vi "Modbus Visa for Solder.vi"(1 "VISA resource name":refnum<visa-resource-name>, 2 "Cmd":string, 3 "TimeOut":bool=TRUE, 4 "Time(0.1)":u32=10, 5 "error in (no error)":errorcluster, 8 "VisaAction":T1(ring)) -> (16 "read string":string, 19 "error out":errorcluster)   [LabVIEW 2019]
uses:
  <vilib>/Instr/_visa.llb/VISA Configure Serial Port (Instr).vi
panel:
  in  "TimeOut 2":bool=TRUE
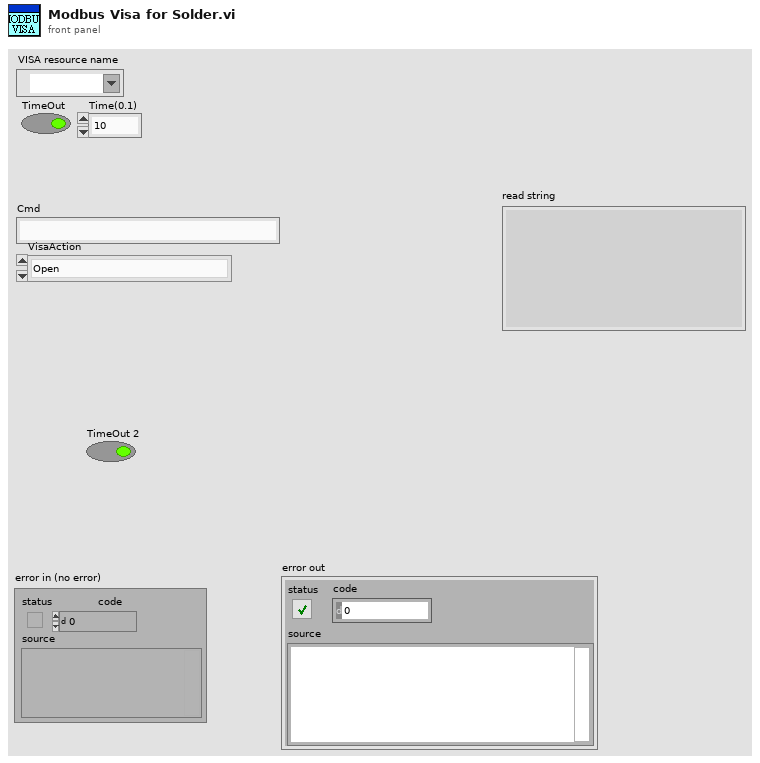
[diagram p1: front panel]
types:
  T1 = enum16{"Open", "Send", "Recieve", "Recieve cmd", "Close"}
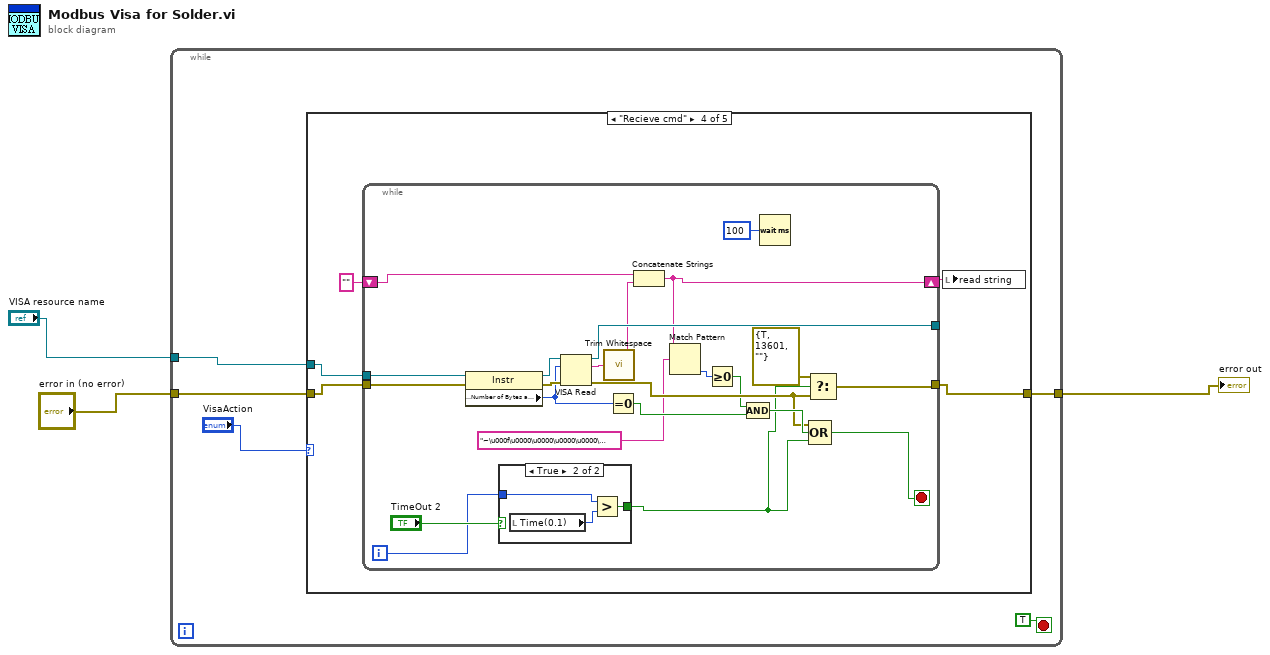
[diagram p0: block diagram]
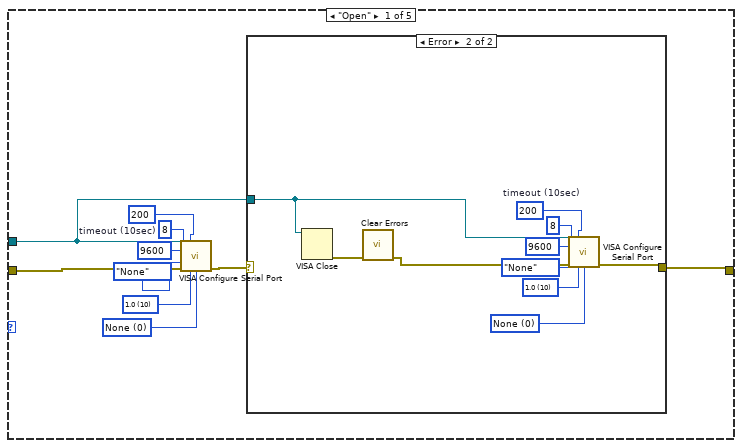
[diagram p2: hidden frame]
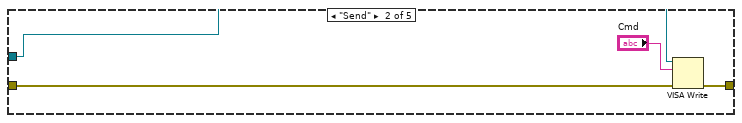
[diagram p4: hidden frame]
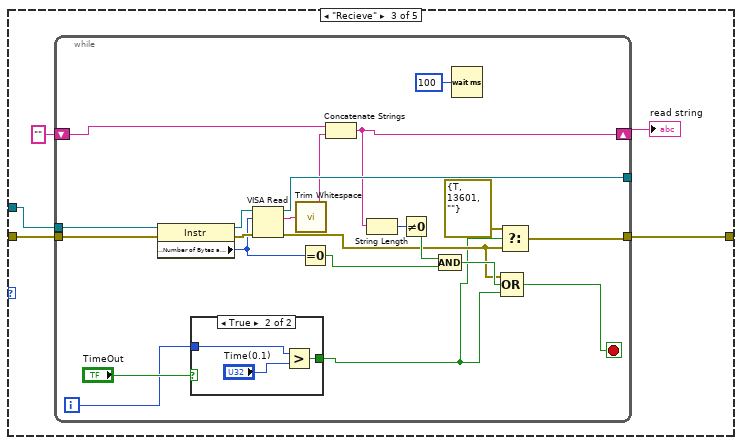
[diagram p5: hidden frame]
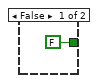
[diagram p6: hidden frame]
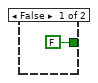
[diagram p7: hidden frame]
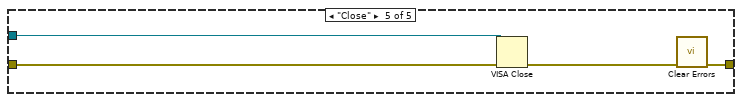
[diagram p8: hidden frame]
diagram:
  n1 = while {
    tunnel: "error in (no error)" -> [w7]
    tunnel: [w8] -> w3
    tunnel: "VISA resource name" -> [w5]
    stop <- TRUE stop-if-true
    n2 = case shown="\"Recieve cmd\"" "VisaAction" {
      tunnel: [w10 w33 w37 w67 w98] -> w8
      tunnel: w7 -> [w18 w32 w38 w65 w99]
      tunnel: w5 -> [w9 w31 w34 w66 w97]
      frame "Open" {
        w13 = u16 0 items=["None", "XON/XOFF", "RTS/CTS", "XON/XOFF & RTS/CTS", "DTR/DSR", "XON/XOFF & DTR/DSR"] ("flow control (0:none)")
        w14 = u16 10 items=["1.0"=10, "1.5"=15, "2.0"=20] ("stop bits (10: 1 bit)")
        w17 = u32 200  # timeout (10sec)
        n3 = call-poly "VISA Configure Serial Port"("VISA resource name"=w9, "timeout (10sec)"=w17, "baud rate (9600)"=u32 9600, "data bits (8)"=u16 8, "parity (0:none)"=enum16{"None", "Odd", "Even", "Mark", "Space"}."None", "error in (no error)"=w18, "stop bits (10: 1 bit)"=w14, "flow control (0:none)"=w13) -> ("error out"=w11:errorcluster)  [unwired: 1 in, 6 out]
        n4 = case shown="Error" w11 {
          selector: w11 -> [w19 _]
          tunnel: [w19 w20] -> w10
          tunnel: w9 -> [_ w21]
          frame No Error {
          }
          frame Error {
            w28 = u16 0 items=["None", "XON/XOFF", "RTS/CTS", "XON/XOFF & RTS/CTS", "DTR/DSR", "XON/XOFF & DTR/DSR"] ("flow control (0:none)")
            w27 = u16 10 items=["1.0"=10, "1.5"=15, "2.0"=20] ("stop bits (10: 1 bit)")
            w24 = u32 200  # timeout (10sec)
            n5 = VISA Close(VISA resource name=w21) -> (error out=w23:errorcluster)  [unwired: 1 in]
            n6 = call <vilib>:"Clear Errors.vi"("error in (no error)"=w23) -> ("error out"=w22:errorcluster)  [unwired: 5 in, 1 out]
            n7 = call-poly "VISA Configure Serial Port"("VISA resource name"=w21, "timeout (10sec)"=w24, "baud rate (9600)"=u32 9600, "data bits (8)"=u16 8, "parity (0:none)"=enum16{"None", "Odd", "Even", "Mark", "Space"}."None", "error in (no error)"=w22, "stop bits (10: 1 bit)"=w27, "flow control (0:none)"=w28) -> ("error out"=w20:errorcluster)  [unwired: 1 in, 6 out]
          }
        }
      }
      frame "Send" {
        n8 = VISA Write(VISA resource name=w31, write buffer="Cmd", error in (no error)=w32) -> (error out=w33:errorcluster)  [unwired: 2 out]
      }
      frame "Recieve" {
        n9 = while {
          tunnel: w38 -> [w58]
          tunnel: [w57] -> _
          tunnel: [w52] -> w37
          shift-right: [w49] -> w36
          shift-left: "" ("trimmed string") -> [w55]
          tunnel: w34 -> [w39]
          i -> [w41]
          stop <- w53 stop-if-true
          n10 = property class="Instr"(reference=w39, error in=w58) -> (reference out=w59:refnum<visa-resource-name>, error out=w60:errorcluster, "Serial Settings:Number of Bytes at Serial Port"=w42:u32)
          n11 = case shown="True" "TimeOut" {
            tunnel: w41 -> [_ w64]
            tunnel: [FALSE w62] -> w40
            frame False {
            }
            frame True {
              n12 = Greater?(x=w64, y="Time(0.1)") -> (0:w62:bool)
            }
          }
          n13 = VISA Read(VISA resource name=w59, byte count=w42, error in (no error)=w60) -> (VISA resource name out=w57:refnum<visa-resource-name>, read buffer=w44:string, error out=w45:errorcluster)  [unwired: 1 out]
          n14 = call <vilib>:"Trim Whitespace.vi"("string"=w44) -> ("trimmed string"=w56:string)  [unwired: 1 in]
          n15 = Equal To 0?(x=w42) -> (x = 0?=w50:bool)
          n16 = Concatenate Strings(w55, w56) -> (w49:string)
          n17 = String Length(string=w49) -> (length=w48:i32)
          n18 = Not Equal To 0?(x=w48) -> (x != 0?=w47:bool)
          n19 = Compound Arithmetic op=AND(w47, w50) -> (w46:bool)
          n20 = Wait (ms)(milliseconds to wait=u32 100) -> ()  [unwired: 1 out]
          n21 = Select(t=errorcluster {"status"=TRUE, "code"=13601, "source"=""}, s=w40, f=w45) -> (s? t:f=w52:errorcluster)
          n22 = Compound Arithmetic op=OR(w45, w46, w40) -> (w53:bool)
        }
        "read string" <- w36
      }
      frame "Recieve cmd" {
        n23 = while {
          tunnel: w65 -> [w90]
          tunnel: [w89] -> _
          tunnel: [w84] -> w67
          shift-right: [w71] -> w68
          shift-left: "" ("trimmed string") -> [w87]
          tunnel: w66 -> [w74]
          i -> [w76]
          stop <- w85 stop-if-true
          n24 = property class="Instr"(reference=w74, error in=w90) -> (reference out=w91:refnum<visa-resource-name>, error out=w92:errorcluster, "Serial Settings:Number of Bytes at Serial Port"=w77:u32)
          n25 = case shown="True" "TimeOut 2" {
            tunnel: w76 -> [_ w96]
            tunnel: [FALSE w95] -> w75
            frame False {
            }
            frame True {
              n26 = local read "Time(0.1)"() -> (w94:u32)
              n27 = Greater?(x=w96, y=w94) -> (0:w95:bool)
            }
          }
          n28 = VISA Read(VISA resource name=w91, byte count=w77, error in (no error)=w92) -> (VISA resource name out=w89:refnum<visa-resource-name>, read buffer=w79:string, error out=w80:errorcluster)  [unwired: 1 out]
          n29 = call <vilib>:"Trim Whitespace.vi"("string"=w79) -> ("trimmed string"=w88:string)  [unwired: 1 in]
          n30 = Equal To 0?(x=w77) -> (x = 0?=w82:bool)
          n31 = Concatenate Strings(w87, w88) -> (w71:string)
          n32 = Match Pattern(string=w71, regular expression="~\u000f\u0000\u0000\u0000\u0000\u0000\u000f~" ("trimmed string")) -> (offset past match=w73:i32)  [unwired: 1 in, 3 out]
          n33 = Greater Or Equal To 0?(x=w73) -> (x >= 0?=w72:bool)
          n34 = Compound Arithmetic op=AND(w72, w82) -> (w81:bool)
          n35 = Wait (ms)(milliseconds to wait=u32 100) -> ()  [unwired: 1 out]
          n36 = Select(t=errorcluster {"status"=TRUE, "code"=13601, "source"=""}, s=w75, f=w80) -> (s? t:f=w84:errorcluster)
          n37 = Compound Arithmetic op=OR(w80, w81, w75) -> (w85:bool)
        }
        n38 = local write "read string"(w68) -> ()
      }
      frame "Close" {
        n39 = VISA Close(VISA resource name=w97, error in (no error)=w99) -> (error out=w100:errorcluster)
        n40 = call <vilib>:"Clear Errors.vi"("error in (no error)"=w100) -> ("error out"=w98:errorcluster)  [unwired: 5 in, 1 out]
      }
    }
  }
  "error out" <- w3
